vi "DAQmx_AOtest.vi"() -> ()   [LabVIEW 2020]
uses:
  Realization/NI Analog Output/NI Analog Output.lvclass
  Realization/NI Analog Output/TypeDefs/Channel Config.ctl
  Realization/NI Analog Output/TypeDefs/Output Config.ctl
  Realization/NI Analog Output/TypeDefs/Timing Config.ctl
  Realization/NI Analog Output/TypeDefs/Trigger Config.ctl
panel:
  out "self-cal":variant
  out "self-test":variant
  out "error out":errorcluster
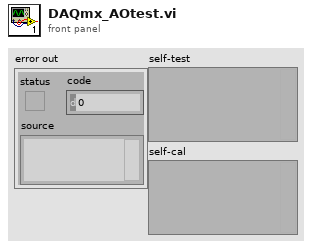
[diagram p1: front panel]
types:
  T1 = typedef "Output Config.ctl" = cluster{"data":variant, "auto start":bool, "regeneration":bool}
  T2 = typedef "Channel Config.ctl" = cluster{"physical channels":string, "maximum value":dbl, "minimum value":dbl, "output terminal configuration":i32, "units":i32}
  T3 = typedef "Trigger Config.ctl" = cluster{"trigger type":string, "source":string, "slope":i32, "analog level":dbl, "analog hysteresis":dbl}
  T4 = typedef "Timing Config.ctl" = cluster{"sample mode":i32, "samples per channel":i32, "rate":dbl, "source":string, "active edge":i32}
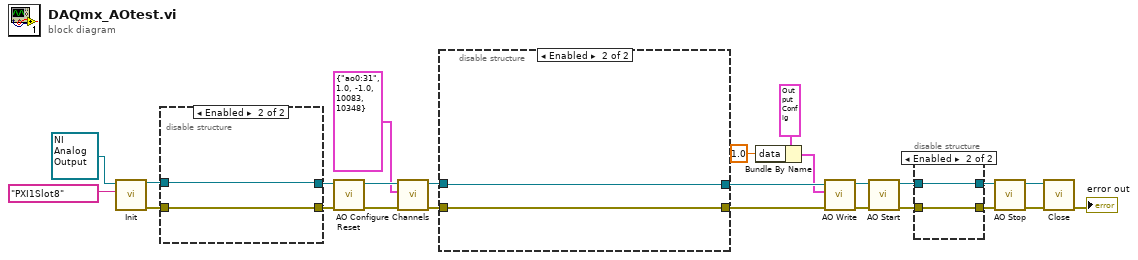
[diagram p0: block diagram]
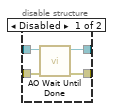
[diagram p2: hidden frame]
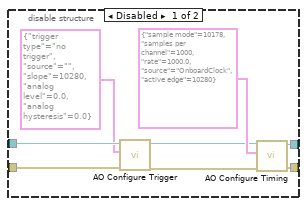
[diagram p3: hidden frame]
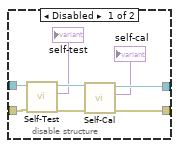
[diagram p4: hidden frame]
diagram:
  n1 = call-dynamic "Init.vi"("Params"="PXI1Slot8", "DAQmx Base in"=refnum<class "NI Analog Output.lvclass"> refnum ("NI DAQmx.lvlib:NI Analog Output.lvclass")) -> ("error out"=w25:errorcluster, "DAQmx Base out"=w24:refnum<class "NI Analog Output.lvclass">)  [unwired: 8 in]
  n2 = disable-structure shown="Enabled" {
    disable-tunnel: w25 -> [w33 w34]
    disable-tunnel: w24 -> [w32 w35]
    disable-tunnel: [w29 w35] -> w23
    disable-tunnel: [w28 w34] -> w22
    frame Disabled {
      n3 = call-dynamic "Self-Test.vi"("error in (no error)"=w33, "DAQmx Base in"=w32) -> ("error out"=w30:errorcluster, "Result"=→"self-test":variant, "DAQmx Base out"=w31:refnum<class "NI Analog Output.lvclass">)  [unwired: 7 in]
      n4 = call-dynamic "Self-Cal.vi"("error in (no error)"=w30, "DAQmx Base in"=w31) -> ("error out"=w28:errorcluster, "Result"=→"self-cal":variant, "DAQmx Base out"=w29:refnum<class "NI Analog Output.lvclass">)  [unwired: 7 in]
    }
    frame Enabled {
    }
  }
  n5 = call-dynamic "Reset.vi"("error in (no error)"=w22, "DAQmx Base in"=w23) -> ("error out"=w18:errorcluster, "DAQmx Base out"=w17:refnum<class "NI Analog Output.lvclass">)  [unwired: 8 in]
  n6 = call-dynamic "AO Configure Channels.vi"("error in (no error)"=w18, "Params"=T2 {"physical channels"="ao0:31", "maximum value"=1.0, "minimum value"=-1.0, "output terminal configuration"=10083, "units"=10348} ("Channel Config"), "NI Analog Output in"=w17) -> ("error out"=w2:errorcluster, "NI Analog Output out"=w1:refnum<class "NI Analog Output.lvclass">)  [unwired: 7 in]
  n7 = disable-structure shown="Enabled" {
    disable-tunnel: [w43 w44] -> w7
    disable-tunnel: [w42 w45] -> w6
    disable-tunnel: w2 -> [w40 w45]
    disable-tunnel: w1 -> [w39 w44]
    frame Disabled {
      n8 = call-dynamic "AO Configure Trigger.vi"("error in (no error)"=w40, "Params"=T3 {"trigger type"="no trigger", "source"="", "slope"=10280, "analog level"=0.0, "analog hysteresis"=0.0} ("Cluster"), "NI Analog Output in"=w39) -> ("error out"=w37:errorcluster, "NI Analog Output out"=w38:refnum<class "NI Analog Output.lvclass">)  [unwired: 7 in]
      n9 = call-dynamic "AO Configure Timing.vi"("error in (no error)"=w37, "Params"=T4 {"sample mode"=10178, "samples per channel"=1000, "rate"=1000.0, "source"="OnboardClock", "active edge"=10280} ("Timing Config"), "NI Analog Output in"=w38) -> ("error out"=w42:errorcluster, "NI Analog Output out"=w43:refnum<class "NI Analog Output.lvclass">)  [unwired: 7 in]
    }
    frame Enabled {
    }
  }
  n10 = Bundle By Name(cluster=T1 {"data"=variant, "auto start"=FALSE, "regeneration"=TRUE} ("Output config"), "data"=1.0) -> (w4:T1)
  n11 = call-dynamic "AO Write.vi"("error in (no error)"=w6, "Params"=w4, "NI Analog Output in"=w7) -> ("error out"=w10:errorcluster, "NI Analog Output out"=w9:refnum<class "NI Analog Output.lvclass">)  [unwired: 7 in]
  n12 = call-dynamic "AO Start.vi"("error in (no error)"=w10, "NI Analog Output in"=w9) -> ("error out"=w12:errorcluster, "NI Analog Output out"=w14:refnum<class "NI Analog Output.lvclass">)  [unwired: 8 in]
  n13 = disable-structure shown="Enabled" {
    disable-tunnel: w14 -> [w49 w51]
    disable-tunnel: [w48 w51] -> w13
    disable-tunnel: w12 -> [w47 w50]
    disable-tunnel: [w46 w50] -> w11
    frame Disabled {
      n14 = call-dynamic "AO Wait Until Done.vi"("error in (no error)"=w47, "NI Analog Output in"=w49) -> ("error out"=w46:errorcluster, "NI Analog Output out"=w48:refnum<class "NI Analog Output.lvclass">)  [unwired: 8 in]
    }
    frame Enabled {
    }
  }
  n15 = call-dynamic "AO Stop.vi"("error in (no error)"=w11, "NI Analog Output in"=w13) -> ("error out"=w15:errorcluster, "NI Analog Output out"=w16:refnum<class "NI Analog Output.lvclass">)  [unwired: 8 in]
  n16 = call-dynamic "Close.vi"("error in (no error)"=w15, "DAQmx Base in"=w16) -> ("error out"=→"error out":errorcluster)  [unwired: 8 in, 1 out]
